vi "get_current_set_low_limit.vi"(8 "error in":errorcluster, 11 "VISA resource name":refnum<visa-resource-name>="COM1") -> (0 "error out":errorcluster, 3 "VISA resource name out":refnum<visa-resource-name>)   [LabVIEW 2020]
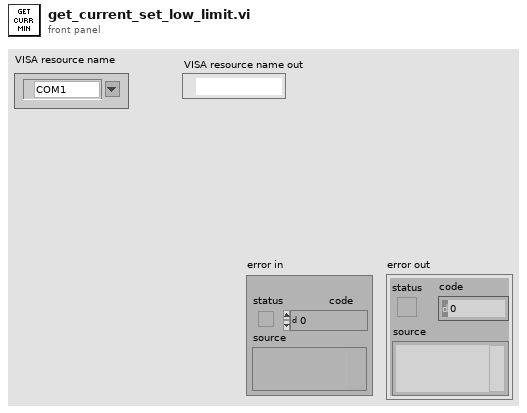
[diagram p1: front panel]
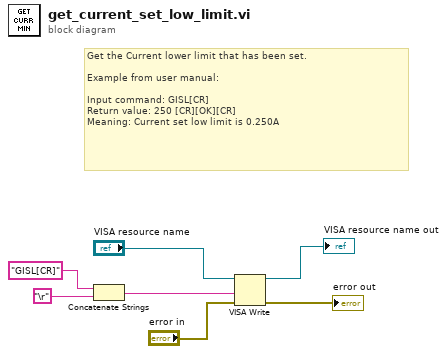
[diagram p0: block diagram]
diagram:
  # "Get the Current lower limit that has been set.\n\nExample from user manual:\n\nInput command: GISL[CR]\nReturn value: 250 [CR][OK][CR]\nMeaning: Current set low limit is 0.250A"
  n1 = Concatenate Strings("GISL[CR]" ("Command"), "\r") -> (w4:string)
  n2 = VISA Write(VISA resource name="VISA resource name", write buffer=w4, error in (no error)="error in") -> (VISA resource name out=→"VISA resource name out":refnum<visa-resource-name>, error out=→"error out":errorcluster)  [unwired: 1 out]
